vi "Password encryption.vi"(6 "error in (no error)":errorcluster, 8 "Key":string, 9 "Password":string) -> (0 "error out":errorcluster, 3 "Output text":string)   [LabVIEW 2009]
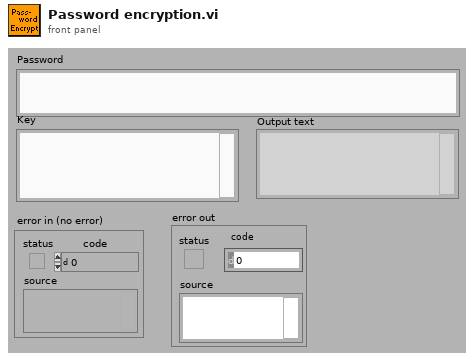
[diagram p1: front panel]
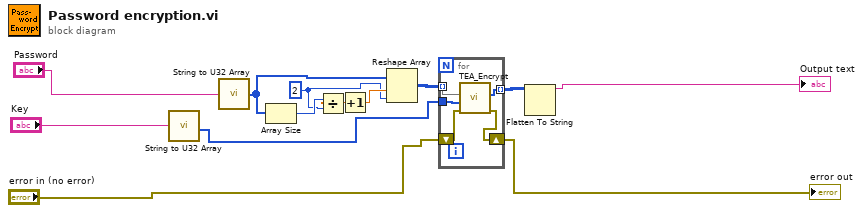
[diagram p0: block diagram]
diagram:
  w3 = 2 ("dimension size")
  n1 = call "String to U32 Array.vi"("string"="Key") -> ("Array"=w10:u32[])
  n2 = call "String to U32 Array.vi"("string"="Password") -> ("Array"=w5:u32[])
  n3 = Array Size(array=w5) -> (size(s)=w9:i32)
  n4 = Divide(x=w9, y=w3) -> (x/y=w8:dbl)
  n5 = Increment(x=w8) -> (x+1=w4:dbl)
  n6 = Reshape Array(w5, w4, w3) -> (w7:u32[][])
  n7 = for {
    tunnel: w10 -> [w18]
    tunnel: [w17] -> w6 mode=indexing
    tunnel: w7 -> [w16] mode=indexing
    shift-right: [w14] -> w1
    shift-left: "error in (no error)" -> [w15]
    n8 = call "TEA_Encrypt.vi"("error in (no error)"=w15, "k"=w18, "V"=w16) -> ("error out"=w14:errorcluster, "Y"=w17:u32[])  [unwired: 7 out]
  }
  "error out" <- w1
  n9 = Flatten To String(anything=w6) -> (data string=→"Output text":string)  [unwired: 1 in, 4 out]
